vi "Send CMD.vi"(8 "error in":errorcluster, 10 "CMD In":string, 11 "Vaisala in":refnum<class "FPGA Vaisala.lvclass">) -> (0 "error out":errorcluster, 3 "Vaisala out":refnum<class "FPGA Vaisala.lvclass">)   [LabVIEW 2015, in "FPGA Vaisala.lvclass"]
uses:
  FPGA Vaisala.lvclass
  FPGA Vaisala.lvclass/FPGA Vaisala.ctl
  <vilib>/Utility/error.llb/Error Cluster From Error Code.vi
  <vilib>/rvi/errors/niLvFpgaAdjustHostInterfaceError.vi
  <vilib>/RVI Host/nirviSupport.llb/nirviErrorClusterFromErrorCode.vi
  <vilib>/rvi/interface/nirviReadWriteControl/nirviReadWriteControl.xnode
  <vilib>/rvi/interface/nirviMethod/nirviMethod.xnode
  NiFpgaLv.dll
  <vilib>/FPGAPlugInAG/cRIO-9081/niLvFpga_AcknowledgeIrq_cRIO-9081.vi
  <vilib>/rvi/interface/nirviMethod/StockFPGA_InlinedMethodWaitForSingleIRQ.vi
  <vilib>/FPGAPlugInAG/cRIO-9081/niLvFpga_WaitOnIrq_cRIO-9081.vi
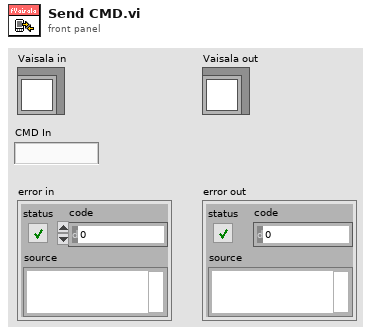
[diagram p1: front panel]
types:
  T1 = enum16{"Port 1", "Port 2", "Port 3", "Port 4", "None"}
  T2 = cluster{"Data":u8[], "NumBytes":i32, "RS485_Cmd":enum16{"Read", "Write", "Idle"}, "New":bool, "Port":enum16{"Port 1", "Port 2", "Port 3", "Port 4", "None"}, "Timeout (ms)":i32}
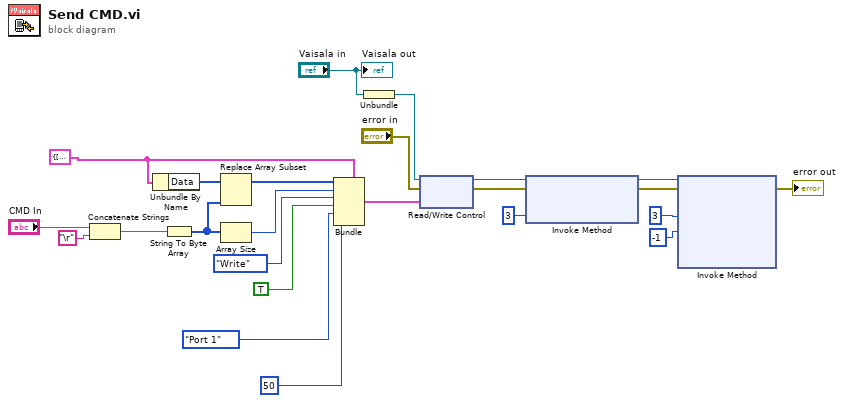
[diagram p0: block diagram]
diagram:
  w5 = T2 {"Data"=[0, 0, 0, 0, 0, 0, 0, 0, 0, 0, 0, 0, 0, 0, 0, 0, 0, 0, 0, 0, 0, 0, 0, 0, 0, 0, 0, 0, 0, 0, 0, 0, 0, 0, 0, 0, 0, 0, 0, 0, 0, 0, 0, 0, 0, 0, 0, 0, 0, 0, 0, 0, 0, 0, 0, 0, 0, 0, 0, 0, 0, 0, 0, 0, 0, 0, 0, 0, 0, 0, 0, 0, 0, 0, 0, 0, 0, 0, 0, 0, 0, 0, 0, 0, 0, 0, 0, 0, 0, 0, 0, 0, 0, 0, 0, 0, 0, 0, 0, 0], "NumBytes"=0, "RS485_Cmd"=enum."Read", "New"=FALSE, "Port"=enum."Port 1", "Timeout (ms)"=0} ("Input")
  n1 = Concatenate Strings("CMD In", "\r") -> (w23:string)
  n2 = Unbundle By Name(w5) -> ("Data"=w22:u8[])
  n3 = String To Byte Array(string=w23) -> (unsigned byte array=w21:u8[])
  n4 = Replace Array Subset(array=w22, new element=w21) -> (w20:u8[])  [unwired: 1 in]
  n5 = Array Size(array=w21) -> (size(s)=w24:i32)
  n6 = Bundle(cluster=w5, "Data"=w20, "NumBytes"=w24, "RS485_Cmd"=enum16{"Read", "Write", "Idle"}."Write", "New"=TRUE ("New Message"), "Port"=T1."Port 1", "Timeout (ms)"=50) -> (w2:T2)
  n7 = Unbundle("Vaisala in") -> (w18:refnum<k20>)
  n8 = xnode "Read/Write Control"("FPGA VI Reference In"=w18, "error in"="error in", "Input"=w2) -> ("FPGA VI Reference Out"=w9:refnum<k20>, "error out"=w7:errorcluster)
  n9 = xnode "Invoke Method"("FPGA VI Reference In"=w9, "error in"=w7, "IRQ Number(s)"=3) -> ("FPGA VI Reference Out"=w13:refnum<k20>, "error out"=w12:errorcluster)
  n10 = xnode "Invoke Method"("FPGA VI Reference In"=w13, "error in"=w12, "IRQ Number(s)"=3, "Timeout (ms)"=-1) -> ("error out"=→"error out":errorcluster)  [unwired: 3 out]
  "Vaisala out" <- "Vaisala in"
